vi "Set HSDIO Voltage Level.vi"(7 "Acq_Logic Family":T1=81 items=["5.0V Logic"=5, "3.3V Logic"=6, "2.5V Logic"=7, "1.8V Logic"=8, "1.5V Logic"=80, "1.2V Logic"=81], 8 "Low Level":dbl format="%.2p", 9 "High Level":dbl=1.8 format="%.2p", 10 "Pins":string[](array[string]), 11 "Semiconductor Module Context":T2) -> (0 "error out":errorcluster)   [LabVIEW 2013]
uses:
  <vilib>/NI_TestStand_SemiconductorModule/NI_TestStand_Semiconductor_Module.lvlibp/PinMap/General/SemiconductorModuleContext.ctl
  <instrlib>/niHSDIO/niHSDIO.llb/niHSDIO_ctl Voltage Logic Family Values (Ring).ctl
  <vilib>/NI_TestStand_SemiconductorModule/NI_TestStand_Semiconductor_Module.lvlibp/PinMap/HSDIO/PinsToNIHSDIOSessions.vi
  <instrlib>/niHSDIO/niHSDIO.llb/niHSDIO Configure Data Voltage Custom Levels.vi
  <instrlib>/niHSDIO/niHSDIO.llb/niHSDIO Configure Data Voltage Logic Family.vi
  <vilib>/NI_TestStand_SemiconductorModule/NI_TestStand_Semiconductor_Module.lvlibp
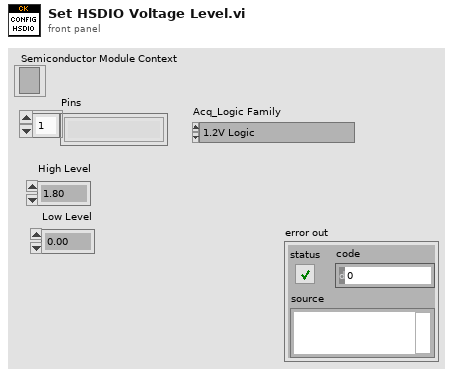
[diagram p1: front panel]
types:
  T1 = typedef "niHSDIO_ctl Voltage Logic Family Values (Ring).ctl" = i32
  T2 = typedef "NI_TestStand_Semiconductor_Module.lvlibp/SemiconductorModuleContext.ctl" = refnum<k7>
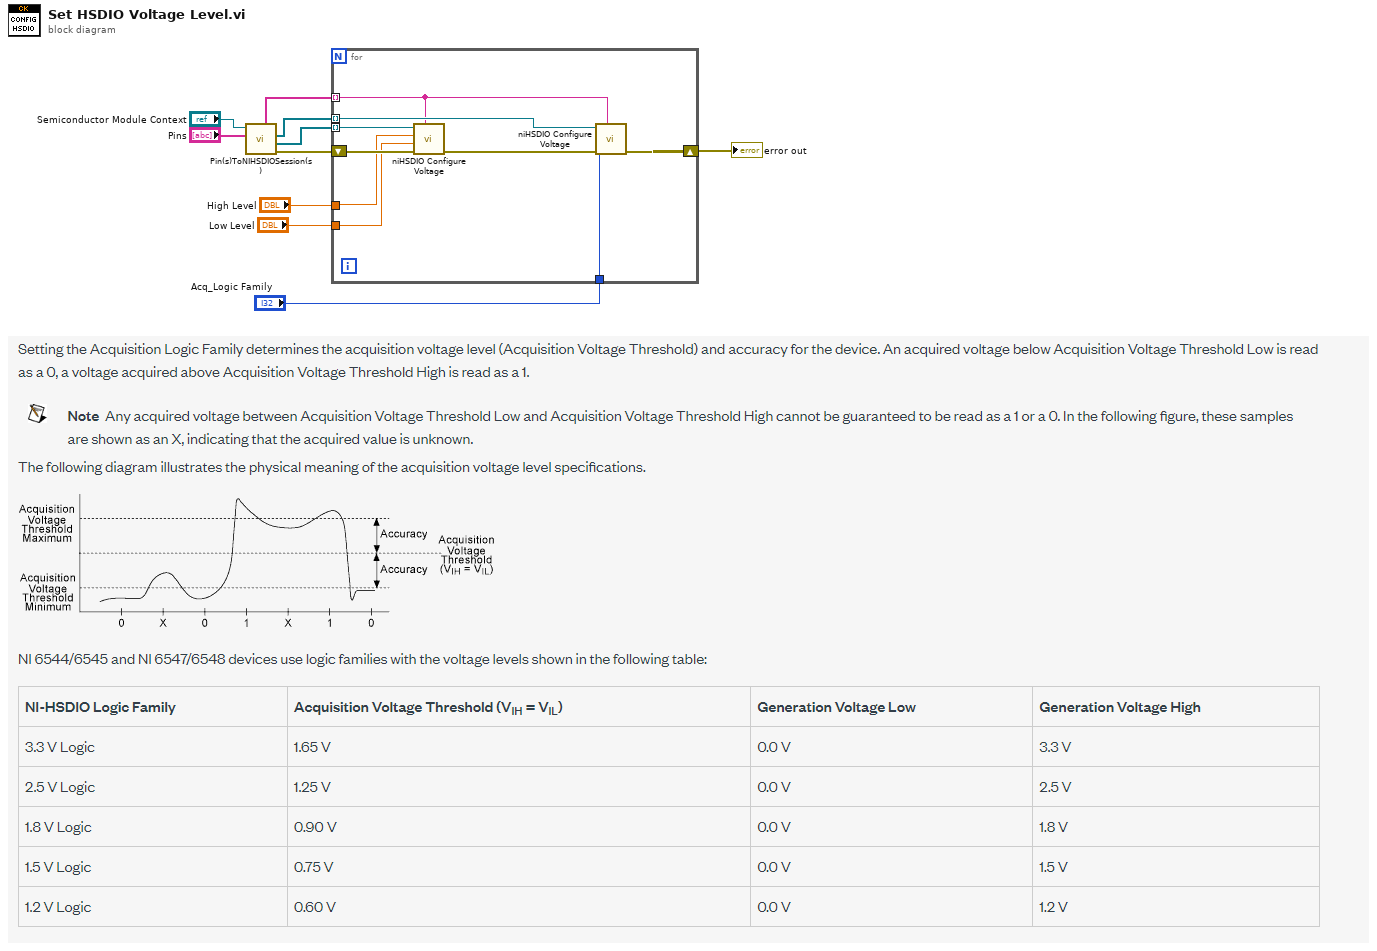
[diagram p0: block diagram]
diagram:
  n1 = call-poly <vilib>:"Pin(s)ToNIHSDIOSession(s).vi"("Pins"="Pins", "Semiconductor Module Context"="Semiconductor Module Context") -> ("error out"=w10:errorcluster, "Generation Sessions"=w8:refnum<k15>[], "Acquisition Sessions"=w2:refnum<k15>[], "Channel Lists"=w9:string[])  [unwired: 4 in, 2 out]
  n2 = for {
    shift-right: [w17] -> w6
    shift-left: w10 -> [w19]
    tunnel: w9 -> [w14] mode=indexing
    tunnel: w8 -> [w18] mode=indexing
    tunnel: "High Level" -> [w13]
    tunnel: "Low Level" -> [w12]
    tunnel: w2 -> [w16] mode=indexing
    tunnel: "Acq_Logic Family" -> [w11]
    n3 = call-poly <instrlib>:"niHSDIO Configure Voltage.vi"("channel list (all:\"\")"=w14, "error in (no error)"=w19, "low level (0.00 volts)"=w12, "high level (3.30 volts)"=w13, "instrument handle"=w18) -> ("error out"=w15:errorcluster)  [unwired: 5 in, 1 out]
    n4 = call-poly <instrlib>:"niHSDIO Configure Voltage.vi"("channel list (all:\"\")"=w14, "error in (no error)"=w15, "logic family (3.3V logic)"=w11, "instrument handle"=w16) -> ("error out"=w17:errorcluster)  [unwired: 6 in, 1 out]
  }
  "error out" <- w6
